vi "TEST - Get Cluster Elements TDs.vi"(8 "error in (no error)":errorcluster) -> (0 "error out":errorcluster, 2 "pass":bool)   [LabVIEW 2020, in "test_openg_array.lvlib"]
uses:
  test_openg_array.lvlib
  <userlib>/_OpenG.lib/error/error.llb/openg_error.lvlib
  source/library/openg_variant.lvlib
panel:
  out "Failures":T1(array[cluster])
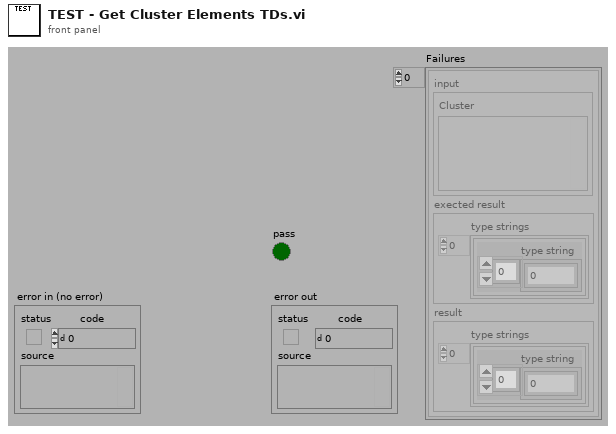
[diagram p1: front panel]
types:
  T1 = cluster{"input":cluster{"Cluster":variant}, "exected result":cluster{"type strings":cluster{"type string":i16[]}[]}, "result":cluster{"type strings":cluster{"type string":i16[]}[]}}[]
  T2 = cluster{"input":cluster{"Cluster":variant}, "exected result":cluster{"type strings":cluster{"type string":i16[]}[]}, "result":cluster{"type strings":cluster{"type string":i16[]}[]}}
  T3 = cluster{"type strings":cluster{"type string":i16[]}[]}
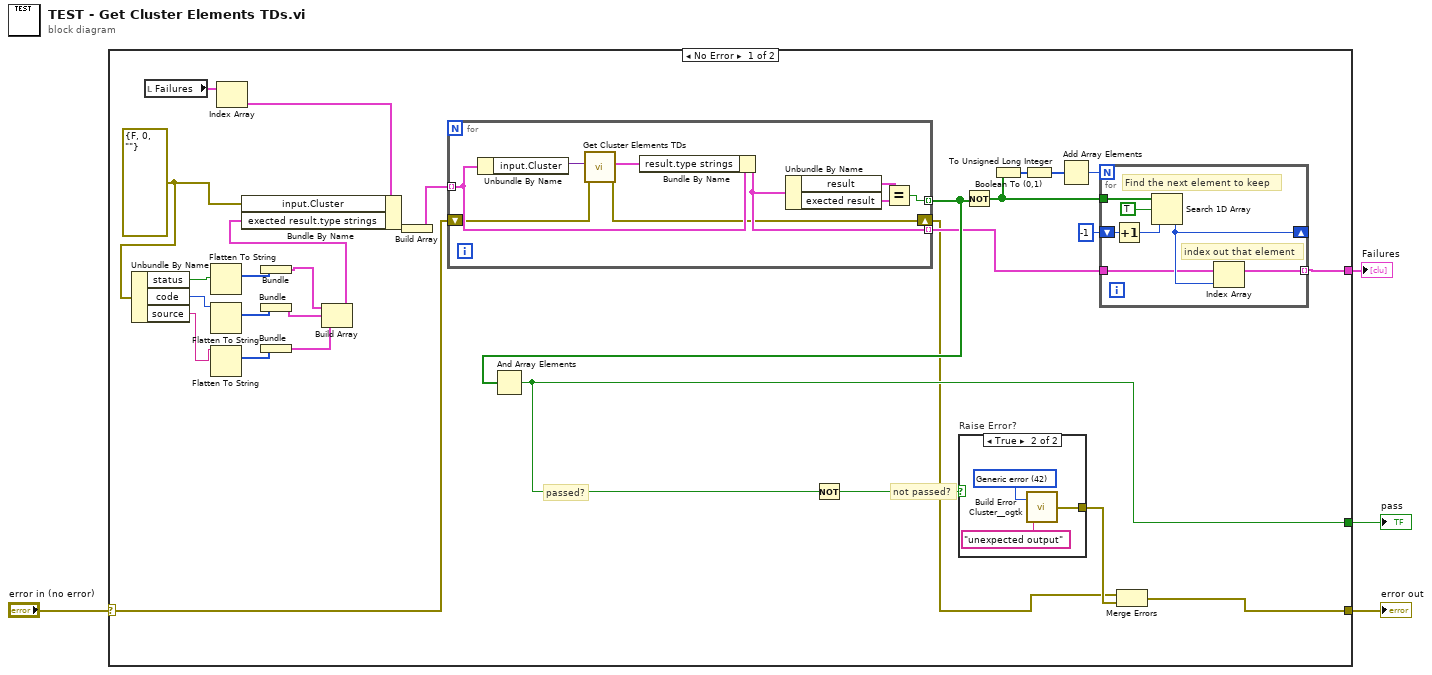
[diagram p0: block diagram]
diagram:
  n1 = case shown="No Error" "error in (no error)" {
    selector: "error in (no error)" -> [w19 w53]
    tunnel: [w30 _] -> w4
    tunnel: [w33 w53] -> w2
    tunnel: [w22 _] -> w1
    frame No Error {
      w15 = errorcluster {"status"=FALSE, "code"=0, "source"=""} ("error in (no error)")
      # "not passed?"
      # "passed?"
      n2 = Unbundle By Name(w15) -> ("status"=w14:bool, "code"=w13:i32, "source"=w12:string)
      n3 = local read "Failures"() -> (w17:T1)
      n4 = Flatten To String(anything=w14) -> (type string=w11:i16[])  [unwired: 3 in, 2 out]
      n5 = Flatten To String(anything=w13) -> (type string=w9:i16[])  [unwired: 3 in, 2 out]
      n6 = Flatten To String(anything=w12) -> (type string=w10:i16[])  [unwired: 3 in, 2 out]
      n7 = Index Array(array=w17) -> (element=w16:T2)  [unwired: 1 in]
      n8 = Bundle("type string"=w11) -> (w6:cluster{"type string":i16[]})  [unwired: 1 in]
      n9 = Bundle("type string"=w9) -> (w7:cluster{"type string":i16[]})  [unwired: 1 in]
      n10 = Bundle("type string"=w10) -> (w8:cluster{"type string":i16[]})  [unwired: 1 in]
      n11 = Build Array(w6, w7, w8) -> (w5:cluster{"type string":i16[]}[])
      n12 = Bundle By Name(cluster=w16, "input.Cluster"=w15, "exected result.type strings"=w5) -> (w21:T2)
      n13 = Build Array(w21) -> (w20:T1)
      n14 = for {
        tunnel: w20 -> [w48] mode=indexing
        tunnel: [w49] -> w24 mode=indexing
        tunnel: [w47] -> w23 mode=indexing
        shift-right: [w42] -> w18
        shift-left: w19 -> [w43]
        n15 = Unbundle By Name(w48) -> ("input.Cluster"=w44:variant)
        n16 = call "Get Cluster Elements TDs.vi"("error in (no error)"=w43, "Cluster"=w44) -> ("error out"=w42:errorcluster, "type strings"=w41:cluster{"type string":i16[]}[])  [unwired: 8 in]
        n17 = Bundle By Name(cluster=w48, "result.type strings"=w41) -> (w47:T2)
        n18 = Unbundle By Name(w47) -> ("result"=w46:T3, "exected result"=w45:T3)
        n19 = Equal?(x=w46, y=w45) -> (x = y?=w49:bool)
      }
      n20 = And Array Elements(Boolean array=w24) -> (logical AND=w30:bool)
      n21 = Not(x=w30) -> (.not. x?=w31:bool)
      n22 = case "Raise Error?" shown="True" w31 {
        tunnel: [_ w50] -> w32
        frame False {
        }
        frame True {
          w51 = 42 items=["No error", "Argument error", "Memory is full", "Out of zone", "End of file", "File already open", "Generic file I/O error", "File not found", "File permission error", "Disk is full", "Duplicate path", "Too many files open", "System feature not enabled", "Resource file not found", "Cannot add resource", "Resource not found", "Image not found", "Image memory error", "Pen does not exist", "Config type invalid", "Config token not found", "Config parse error", "Config memory error", "Bad external code format", "Bad external code offset", "External code not present", "Null window", "Destroy window error", "Null menu", "Print aborted", "Bad print record", "Print driver error", "Windows error during printing", "Memory error during printing", "Print dialog error", "Generic print error", "Invalid device refnum", "Device not found", "Device parameter error", "Device unit error", "Cannot open device", "Device call aborted", "Generic error", "Cancelled by user", "Object ID too low", "Object ID too high", "Object not in heap", "Unknown heap", "Unknown object (invalid DefProc)", "Unknown object (DefProc not in table)", "Message out of range", "Invalid (null) method", "Unknown message", "Manager call not supported", "Bad address", "Network operation in progress", "Network operation timed out", "Connection is busy", "Network attribute not supported", "Network error", "Address in use", "System out of memory", "Connection aborted", "Connection refused", "Not connected", "Already connected", "Connection closed", "Initialization error (interapplication manager)", "Bad occurrence", "Wait on unbound occurrence handler", "Occurrence queue overflow", "Datalog type conflict", "Unused", "Unrecognized type (interapplication manager)", "Memory corrupt", "Failed to make temporary DLL", "Old CIN version", "Drag socket not found", "Failed to load drop-object", "Failed to register OLE object", "Failed to release OLE object", "Format specifier type mismatch", "Unknown format specifier", "Too few format specifiers", "Too many format specifiers", "Scan failed", "Newer CIN version", "Error converting to variant", "Runtime menu error", "Password tampered", "Variant attribute not found", "Incompatible variant data type", "Event data is not available", "Event Store is not present", "Occurrence is not found", "Event Queue is not created", "Event info is not available", "Refnum passed is NULL", "Error retrieving Class GUID", "Error retrieving CoClass GUID", "Error retrieving TypeLib GUID.", "Bad built application magic bytes.", "Specific driver is different from the specific driver associated with the Logical Name.", "There is no session opened to the class driver.", "Max Error", "MAX - Error with config objects", "MAX - Error loading configuration", "MAX - Group not supported"]
          n23 = call <userlib>:"Build Error Cluster__ogtk.vi"("String to Prepend to source (\"\")"="unexpected output" ("String to Prepend to source (\"\")"), "code"=w51) -> ("error out"=w50:errorcluster)
        }
      }
      n24 = Not(x=w24) -> (.not. x?=w26:bool[])
      n25 = Boolean To (0,1)(Boolean=w26) -> (0, 1=w27:i16[])
      n26 = To Unsigned Long Integer(number=w27) -> (unsigned 32bit integer=w25:u32[])
      n27 = Add Array Elements(numeric array=w25) -> (sum=w28:u32)
      n28 = for {
        N: w28 -> [_]
        tunnel: w23 -> [w36]
        tunnel: w26 -> [w40]
        shift-right: [w37] -> _
        shift-left: -1 ("start index (0)") -> [w38]
        tunnel: [w35] -> w22 mode=indexing
        # "index out that element"
        # "Find the next element to keep"
        n29 = Increment(x=w38) -> (x+1=w34:i32)
        n30 = Search 1D Array(1D array=w40, element=TRUE, start index (0)=w34) -> (index of element=w37:i32)
        n31 = Index Array(array=w36, index=w37) -> (element=w35:T2)
      }
      n32 = Merge Errors(w18, w32) -> (w33:errorcluster)
    }
    frame Error {
    }
  }
  "pass" <- w4
  "error out" <- w2
  "Failures" <- w1
